vi "FTW-ScheduledJob-ReadyOrNot.vi"(0 "Scheduled Job Synchronized to System Clock":refnum<class "FTW-ScheduledJob-SyncToSystemClock.lvclass">, 11 "error in":errorcluster) -> (4 "Scheduled Job Synchronized to System Clock out":refnum<class "FTW-ScheduledJob-SyncToSystemClock.lvclass">, 6 "Next Schedule Deadline":u32 format="%d msec", 8 "Next Schedule Active":bool, 10 "Ready to Schedule":bool, 15 "error out":errorcluster)   [LabVIEW 2015, in "FTW-ScheduledJob-SyncToSystemClock.lvclass"]
uses:
  FTW-ScheduledJob-SyncToSystemClock.lvclass
panel:
  # "Inputs"
  # "Outputs"
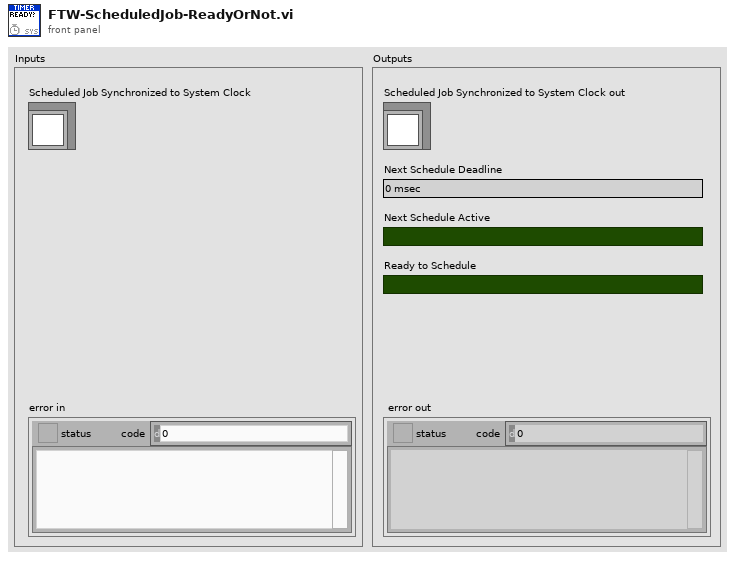
[diagram p1: front panel]
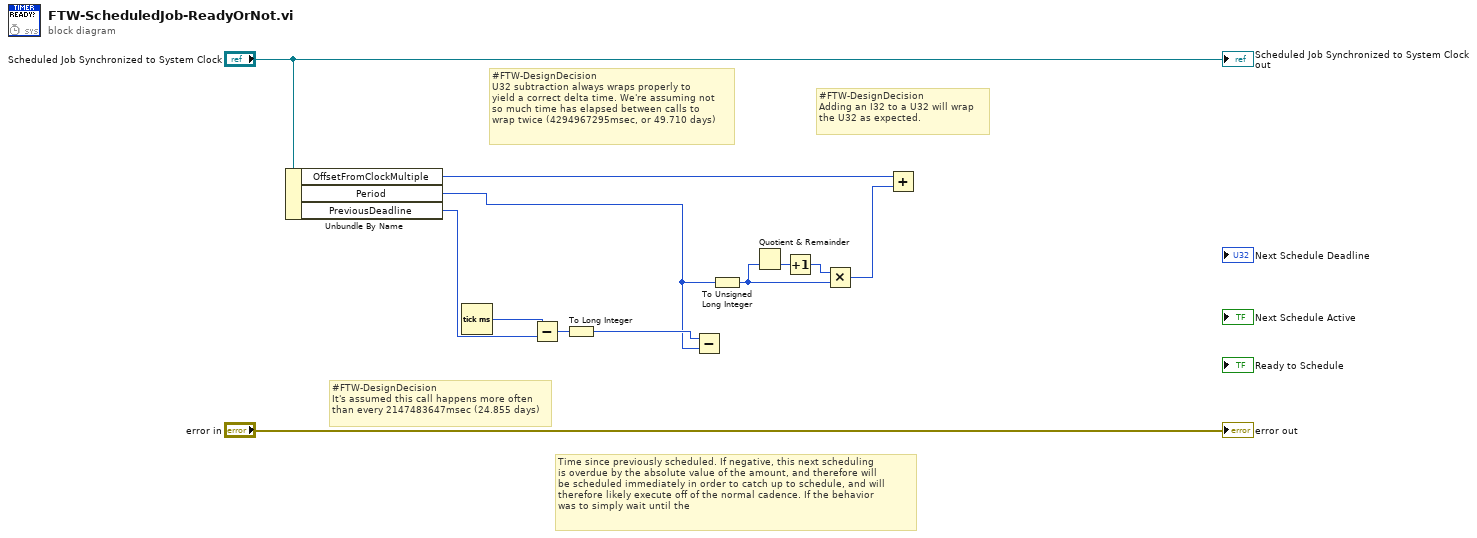
[diagram p0: block diagram]
diagram:
  # "Time since previously scheduled. If negative, this next scheduling\nis overdue by the absolute value of the amount, and therefore will\nbe scheduled immediately in order to catch up to schedule, and will\ntherefore likely execute off of the normal cadence. If the behavior\nwas to simply wait until the"
  # "#FTW-DesignDecision\nU32 subtraction always wraps properly to\nyield a correct delta time. We're assuming not\nso much time has elapsed between calls to\nwrap twice (4294967295msec, or 49.710 days)"
  # "#FTW-DesignDecision\nIt's assumed this call happens more often\nthan every 2147483647msec (24.855 days)"
  # "#FTW-DesignDecision\nAdding an I32 to a U32 will wrap\nthe U32 as expected."
  n1 = Unbundle By Name("Scheduled Job Synchronized to System Clock") -> ("OffsetFromClockMultiple"=w7:i32, "Period"=w1:i32, "PreviousDeadline"=w3:u32)
  n2 = Tick Count (ms)() -> (millisecond timer value=w4:u32)
  n3 = Subtract(x=w4, y=w3) -> (x-y=w5:u32)
  n4 = To Long Integer(number=w5) -> (32bit integer=w2:i32)
  n5 = Subtract(x=w2, y=w1) -> ()  [unwired: 1 out]
  n6 = To Unsigned Long Integer(number=w1) -> (unsigned 32bit integer=w9:u32)
  n7 = Quotient & Remainder(y=w9) -> (x=w8:u32, floor(x/y)=w10:u32)  [unwired: 1 out]
  n8 = Increment(x=w10) -> (x+1=w11:u32)
  n9 = Multiply(x=w11, y=w9) -> (x*y=w6:u32)
  n10 = Add(x=w7, y=w6) -> ()  [unwired: 1 out]
  "Scheduled Job Synchronized to System Clock out" <- "Scheduled Job Synchronized to System Clock"
  "error out" <- "error in"
